vi "XW UV from U1U2 Psi k PN.vi"(0 "U1cal (m/s)":dbl[](array[numeric]), 5 "U2cal (m/s)":dbl[](array[numeric])) -> (3 "U (m/s)":dbl[](array[numeric]), 4 "V (m/s)":dbl[](array[numeric]), 6 "Psi1 (deg)":dbl[](array[numeric]), 8 "Psi2 (deg)":dbl[](array[numeric]), 10 "k1":dbl[](array[numeric]), 14 "Unconverged points (fraction)":dbl, 15 "k2":dbl[](array[numeric]))   [LabVIEW 2011]
uses:
  <vilib>/gmath/NI_Gmath.lvlib
panel:
  out "Checks":dbl[][](graph)
  out "Iters":i32
  in  "maxIter":i32=150
  in  "tol":dbl=1e-06
  # "Paul Nathan 23/04/10"
  # "THIS GRAPH MUST BE RE-ENABLED FROM THE BLOCK DIAGRAM IF NEEDED"
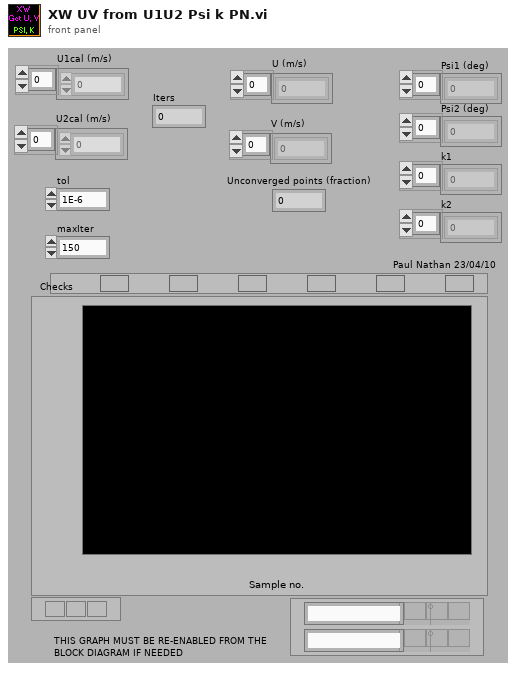
[diagram p1: front panel]
types:
  T1 = typedef "NI_Gmath.lvlib/in_piecewise interp poly control.ctl" = cluster{"x locations":dbl[], "coefficients":dbl[][]}
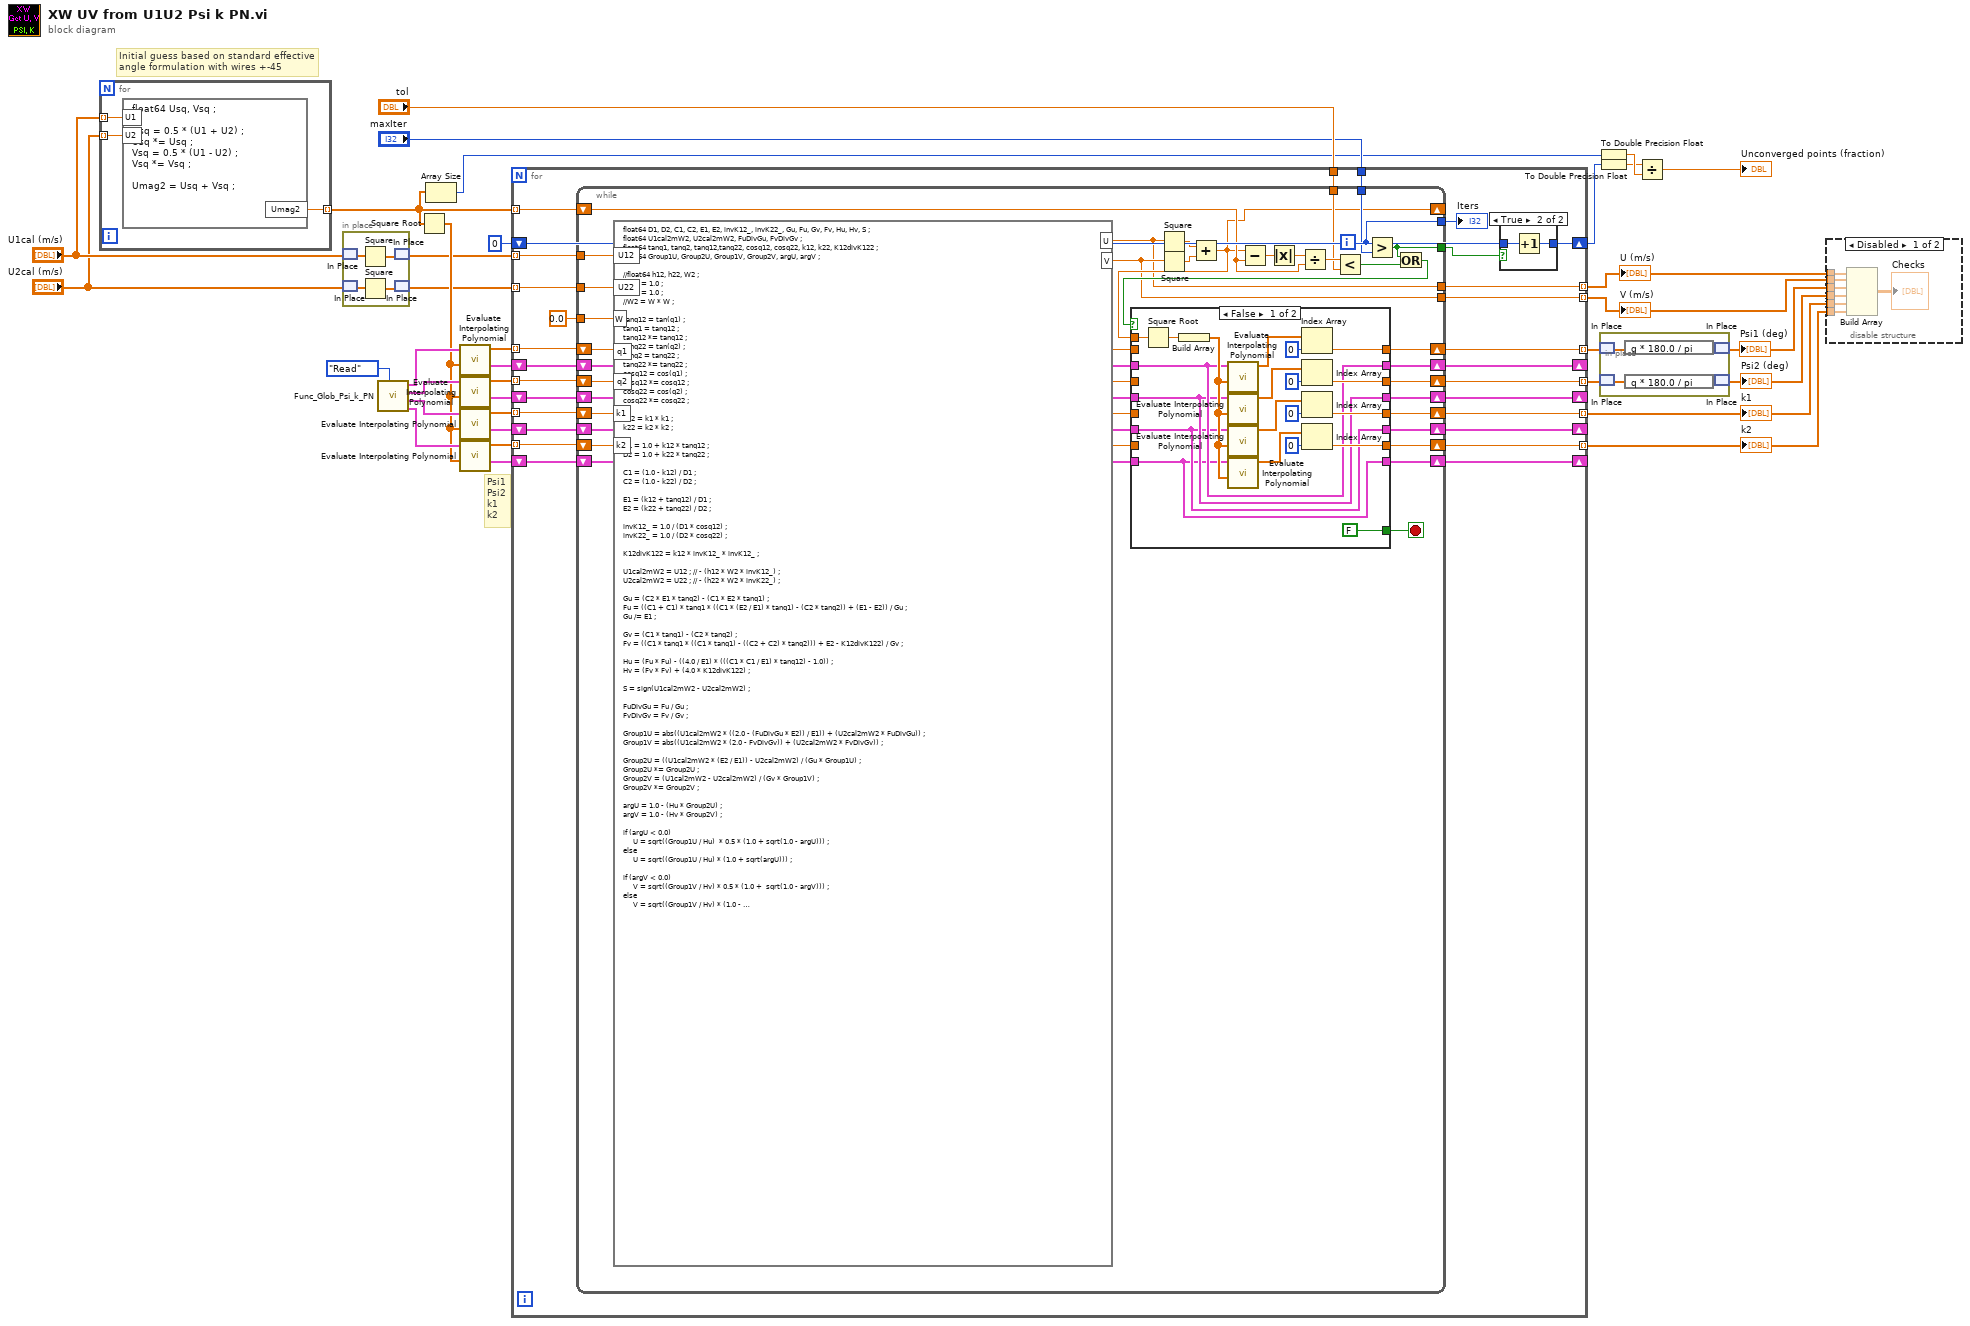
[diagram p0: block diagram]
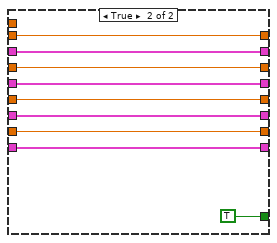
[diagram p4: hidden frame]
diagram:
  # "Initial guess based on standard effective angle formulation with wires +-45"
  # "Psi1\nPsi2\nk1\nk2"
  n1 = for {
    tunnel: "U1cal (m/s)" -> [w34] mode=indexing
    tunnel: "U2cal (m/s)" -> [w33] mode=indexing
    tunnel: [w32] -> w12 mode=indexing
    n2 = formula code="float64 Usq, Vsq ;\n\nUsq = 0.5 * (U1 + U2) ;\nUsq *= Usq ;\nVsq = 0.5 * (U1 - U2) ;\nVsq *= Vsq ;\n\nUmag2 = Usq + Vsq ;"("U1"=w34, "U2"=w33) -> ("Umag2"=w32:dbl)
  }
  n3 = in-place {
    n4 = in-place-match #1("U1cal (m/s)") -> (w37:dbl[])
    n5 = in-place-match #2("U2cal (m/s)") -> (w38:dbl[])
    n6 = Square(x=w37) -> (x^2=w36:dbl[])
    n7 = Square(x=w38) -> (x^2=w35:dbl[])
    n8 = in-place-match #1(w36) -> (w16:dbl[])
    n9 = in-place-match #2(w35) -> (w17:dbl[])
  }
  n10 = call "Func_Glob_Psi_k_PN.vi"("Action"=enum16{"Read", "Write"}."Read") -> ("k2 coeffs OUT"=w27:T1, "k1 coeffs OUT"=w28:T1, "Psi2 coeffs OUT"=w29:T1, "Psi1 coeffs OUT"=w30:T1)  [unwired: 4 in]
  n11 = Square Root(x=w12) -> (sqrt(x)=w20:dbl[])
  n12 = Array Size(array=w12) -> (size(s)=w11:i32)
  n13 = call <vilib>:"Evaluate Interpolating Polynomial.vi"("xi"=w20, "piecewise polynomial"=w30) -> ("yi"=w26:dbl[])  [unwired: 9 out]
  n14 = call <vilib>:"Evaluate Interpolating Polynomial.vi"("xi"=w20, "piecewise polynomial"=w29) -> ("yi"=w25:dbl[])  [unwired: 9 out]
  n15 = call <vilib>:"Evaluate Interpolating Polynomial.vi"("xi"=w20, "piecewise polynomial"=w28) -> ("yi"=w24:dbl[])  [unwired: 9 out]
  n16 = call <vilib>:"Evaluate Interpolating Polynomial.vi"("xi"=w20, "piecewise polynomial"=w27) -> ("yi"=w23:dbl[])  [unwired: 9 out]
  n17 = for {
    tunnel: w16 -> [w48] mode=indexing
    tunnel: w17 -> [w47] mode=indexing
    shift-right: [w58] -> _
    shift-left: w30 -> [w62]
    shift-right: [w57] -> _
    shift-left: w29 -> [w61]
    shift-right: [w56] -> _
    shift-left: w28 -> [w60]
    shift-right: [w55] -> _
    shift-left: w27 -> [w59]
    tunnel: w26 -> [w66] mode=indexing
    tunnel: w25 -> [w65] mode=indexing
    tunnel: w24 -> [w64] mode=indexing
    tunnel: w23 -> [w63] mode=indexing
    tunnel: [w54] -> w7 mode=indexing
    tunnel: [w53] -> w2 mode=indexing
    tunnel: "tol" -> [w52]
    tunnel: "maxIter" -> [w51]
    shift-right: [w39] -> w10
    shift-left: 0 -> [w40]
    tunnel: [w46] -> w18 mode=indexing
    tunnel: [w45] -> w19 mode=indexing
    tunnel: [w44] -> w4 mode=indexing
    tunnel: [w43] -> w3 mode=indexing
    tunnel: w12 -> [w42] mode=indexing
    n18 = while {
      tunnel: w48 -> [w104]
      tunnel: w47 -> [w103]
      shift-right: [w83] -> w46
      shift-left: w66 -> [w79]
      shift-right: [w82] -> w45
      shift-left: w65 -> [w78]
      shift-right: [w81] -> w44
      shift-left: w64 -> [w77]
      shift-right: [w80] -> w43
      shift-left: w63 -> [w76]
      shift-right: [w87] -> w58
      shift-left: w62 -> [w88]
      shift-right: [w86] -> w57
      shift-left: w61 -> [w89]
      shift-right: [w85] -> w56
      shift-left: w60 -> [w90]
      shift-right: [w84] -> w55
      shift-left: w59 -> [w91]
      tunnel: [w73] -> w54
      tunnel: [w74] -> w53
      shift-right: [w75] -> _
      shift-left: w42 -> [w98]
      tunnel: w52 -> [w96]
      tunnel: w51 -> [w95]
      tunnel: 0.0 -> [w72]
      tunnel: [w71] -> w49
      tunnel: [w70] -> w41
      i -> [w71]
      stop <- w92 stop-if-true
      n19 = formula code="float64 D1, D2, C1, C2, E1, E2, invK12_, invK22_, Gu, Fu, Gv, Fv, Hu, Hv, S ;\nfloat64 U1cal2mW2, U2cal2mW2, FuDivGu, FvDivGv ;\nfloat64 tanq1, tanq2, tanq12,tanq22, cosq12, cosq22, k12, k22, K12divK122 ;\nfloat64 Group1U, Group2U, Group1V, Group2V, argU, argV ;\n\n//float64 h12, h22, W2 ;\n//h12 = 1.0 ;\n//h22 = 1.0 ;\n//W2 = W * W ;\n\ntanq12 = tan(q1) ;\ntanq1 = tanq12 ;\ntanq12 *= tanq12 ;\ntanq22 = tan(q2) ;\ntanq2 = tanq22 ;\ntanq22 *= tanq22 ;\ncosq12 = cos(q1) ;\ncosq12 *= cosq12 ;\ncosq22 = cos(q2) ;\ncosq22 *= cosq22 ;\n\nk12 = k1 * k1 ;\nk22 = k2 * k2 ;\n\nD1 = 1.0 + k12 * tanq12 ;\nD2 = 1.0 + k22 * tanq22 ;\n\nC1 = (1.0 - k12) / D1 ;\nC2 = (1.0 - k22) / D2 ;\n\nE1 = (k12 + tanq12) / D1 ;\nE2 = (k22 + tanq22) / D2 ;\n\ninvK12_ = 1.0 / (D1 * cosq12) ;\ninvK22_ = 1.0 / (D2 * cosq22) ;\n\nK12divK122 = k12 * invK12_ * invK12_ ;\n\nU1cal2mW2 = U12 ; // - (h12 * W2 * invK12_) ;\nU2cal2mW2 = U22 ; // - (h22 * W2 * invK22_) ;\n\nGu = (C2 * E1 * tanq2) - (C1 * E2 * tanq1) ;\nFu = ((C1 + C1) * tanq1 * ((C1 * (E2 / E1) * tanq1) - (C2 * tanq2)) + (E1 - E2)) / Gu ;\nGu /= E1 ;\n\nGv = (C1 * tanq1) - (C2 * tanq2) ;\nFv = ((C1 * tanq1 * ((C1 * tanq1) - ((C2 + C2) * tanq2))) + E2 - K12divK122) / Gv ;\n\nHu = (Fu * Fu) - ((4.0 / E1) * (((C1 * C1 / E1) * tanq12) - 1.0)) ;\nHv = (Fv * Fv) + (4.0 * K12divK122) ;\n\nS = sign(U1cal2mW2 - U2cal2mW2) ;\n\nFuDivGu = Fu / Gu ;\nFvDivGv = Fv / Gv ;\n\nGroup1U = abs((U1cal2mW2 * ((2.0 - (FuDivGu * E2)) / E1)) + (U2cal2mW2 * FuDivGu)) ;\nGroup1V = abs((U1cal2mW2 * (2.0 - FvDivGv)) + (U2cal2mW2 * FvDivGv)) ;\n\nGroup2U = ((U1cal2mW2 * (E2 / E1)) - U2cal2mW2) / (Gu * Group1U) ;\nGroup2U *= Group2U ;\nGroup2V = (U1cal2mW2 - U2cal2mW2) / (Gv * Group1V) ;\nGroup2V *= Group2V ;\n\nargU = 1.0 - (Hu * Group2U) ;\nargV = 1.0 - (Hv * Group2V) ;\n\nif (argU < 0.0)\n     U = sqrt((Group1U / Hu)  * 0.5 * (1.0 + sqrt(1.0 - argU))) ;\nelse\n     U = sqrt((Group1U / Hu) * (1.0 + sqrt(argU))) ;\n\nif (argV < 0.0)\n     V = sqrt((Group1V / Hv) * 0.5 * (1.0 +  sqrt(1.0 - argV))) ;\nelse\n     V = sqrt((Group1V / Hv) * (1.0 - sqrt(argV))) ;\n\nif (S<0.0) V = -V ;"("U12"=w104, "U22"=w103, "q1"=w79, "q2"=w78, "k1"=w77, "k2"=w76, "W"=w72) -> ("U"=w73:dbl, "V"=w74:dbl)
      n20 = Square(x=w73) -> (x^2=w102:dbl)
      n21 = Square(x=w74) -> (x^2=w101:dbl)
      n22 = Add(x=w102, y=w101) -> (x+y=w75:dbl)
      n23 = Subtract(x=w75, y=w98) -> (x-y=w100:dbl)
      n24 = Absolute Value(x=w100) -> (abs(x)=w99:dbl)
      n25 = Divide(x=w99, y=w98) -> (x/y=w97:dbl)
      n26 = Less?(x=w97, y=w96) -> (x < y?=w94:bool)
      n27 = Greater?(x=w71, y=w95) -> (0:w70:bool)
      n28 = Or(x=w70, y=w94) -> (x .or. y?=w93:bool)
      n29 = case shown="False" w93 {
        tunnel: w75 -> [w123 _]
        tunnel: [FALSE TRUE] -> w92
        tunnel: w91 -> [w105 w129]
        tunnel: w90 -> [w106 w130]
        tunnel: w89 -> [w107 w131]
        tunnel: w88 -> [w108 w132]
        tunnel: [w108 w132] -> w87
        tunnel: [w107 w131] -> w86
        tunnel: [w106 w130] -> w85
        tunnel: [w105 w129] -> w84
        tunnel: [w119 w128] -> w83
        tunnel: [w115 w127] -> w82
        tunnel: [w111 w126] -> w81
        tunnel: [w109 w125] -> w80
        tunnel: w79 -> [_ w128]
        tunnel: w78 -> [_ w127]
        tunnel: w77 -> [_ w126]
        tunnel: w76 -> [_ w125]
        frame False {
          n30 = Square Root(x=w123) -> (sqrt(x)=w122:dbl)
          n31 = Build Array(w122) -> (w121:dbl[])
          n32 = call <vilib>:"Evaluate Interpolating Polynomial.vi"("xi"=w121, "piecewise polynomial"=w108) -> ("yi"=w118:dbl[])  [unwired: 9 out]
          n33 = call <vilib>:"Evaluate Interpolating Polynomial.vi"("xi"=w121, "piecewise polynomial"=w107) -> ("yi"=w116:dbl[])  [unwired: 9 out]
          n34 = call <vilib>:"Evaluate Interpolating Polynomial.vi"("xi"=w121, "piecewise polynomial"=w106) -> ("yi"=w112:dbl[])  [unwired: 9 out]
          n35 = call <vilib>:"Evaluate Interpolating Polynomial.vi"("xi"=w121, "piecewise polynomial"=w105) -> ("yi"=w110:dbl[])  [unwired: 9 out]
          n36 = Index Array(array=w118, index=0) -> (element=w119:dbl)
          n37 = Index Array(array=w116, index=0) -> (element=w115:dbl)
          n38 = Index Array(array=w112, index=0) -> (element=w111:dbl)
          n39 = Index Array(array=w110, index=0) -> (element=w109:dbl)
        }
        frame True {
        }
      }
    }
    "Iters" <- w49
    n40 = case shown="True" w41 {
      tunnel: w40 -> [w67 w69]
      tunnel: [w67 w68] -> w39
      frame False {
      }
      frame True {
        n41 = Increment(x=w69) -> (x+1=w68:i32)
      }
    }
  }
  "U (m/s)" <- w7
  "V (m/s)" <- w2
  "k1" <- w4
  "k2" <- w3
  n42 = To Double Precision Float(number=w11) -> (double precision float=w9:dbl)
  n43 = To Double Precision Float(number=w10) -> (double precision float=w8:dbl)
  n44 = in-place {
    n45 = in-place-match #3(w18) -> (w135:dbl[])
    n46 = in-place-match #4(w19) -> (w137:dbl[])
    n47 = expression code="q * 180.0 / pi"(w135) -> (w134:dbl[])
    n48 = expression code="q * 180.0 / pi"(w137) -> (w136:dbl[])
    n49 = in-place-match #3(w134) -> (w6:dbl[])
    n50 = in-place-match #4(w136) -> (w5:dbl[])
  }
  "Psi1 (deg)" <- w6
  "Psi2 (deg)" <- w5
  n51 = Divide(x=w8, y=w9) -> (x/y=→"Unconverged points (fraction)":dbl)
  n52 = disable-structure shown="Disabled" {
    disable-tunnel: w7 -> [w144 _]
    disable-tunnel: w6 -> [w143 _]
    disable-tunnel: w5 -> [w142 _]
    disable-tunnel: w4 -> [w141 _]
    disable-tunnel: w3 -> [w140 _]
    disable-tunnel: w2 -> [w139 _]
    frame Disabled {
      n53 = Build Array(w144, w139, w143, w142, w141, w140) -> (→"Checks":dbl[][])
    }
    frame Enabled {
    }
  }
